vi "Dispenser Testing.vi"() -> ()   [LabVIEW 2017]
uses:
  Shared Components/Config Manager Class/Type Definitions/Potting Parameters.ctl
  Shared Components/Gantry Class/Type Definitions/Virtual Modes.ctl
  Shared Components/Gantry Class/Type Definitions/Init_Modes.ctl
  Shared Components/Config Manager Class/Type Definitions/Camera Enum.ctl
  Shared Components/WorkTable Class/Type Definitions/Worktable_Syringe.ctl
  Shared Components/Vec3d Class/Vec3d Class.lvclass
  Shared Components/Config Manager Class/Type Definitions/Potting Surface Type.ctl
  Shared Components/Gantry Class/Gantry Class.lvclass
  Shared Components/SyringeTool Class/SyringeTool Class.lvclass
  Shared Components/WorkTable Class/WorkTable Class.lvclass
panel:
  in  "Virtual Mode":T1=enum."Virtual"
  in  "Type of Potting":enum16{"Long Line", "Line", "Points"}(ring)
  in  "Potting Parameters":T2={"Curing Param A"=0.0, "Curing Param B"=0.0, "Speed Nominal"=0.5, "Time Nominal"=2.0, "Turn-on Time"=0.5, "Turn-off Time"=0.1, "Safe Height Offset"=0.0, "Tip Height"=0.18, "Width of Line"=0.0, "Number of lines"=0.0, "Distance between lines"=0.1}
  in  "stop":bool
  out "Image":T3(plugin-control)
  out "error out":errorcluster
  in  "Config Folder":path=path "C:/Users/Admin/Gantry Purdue/pixel-gantry-control/Config"
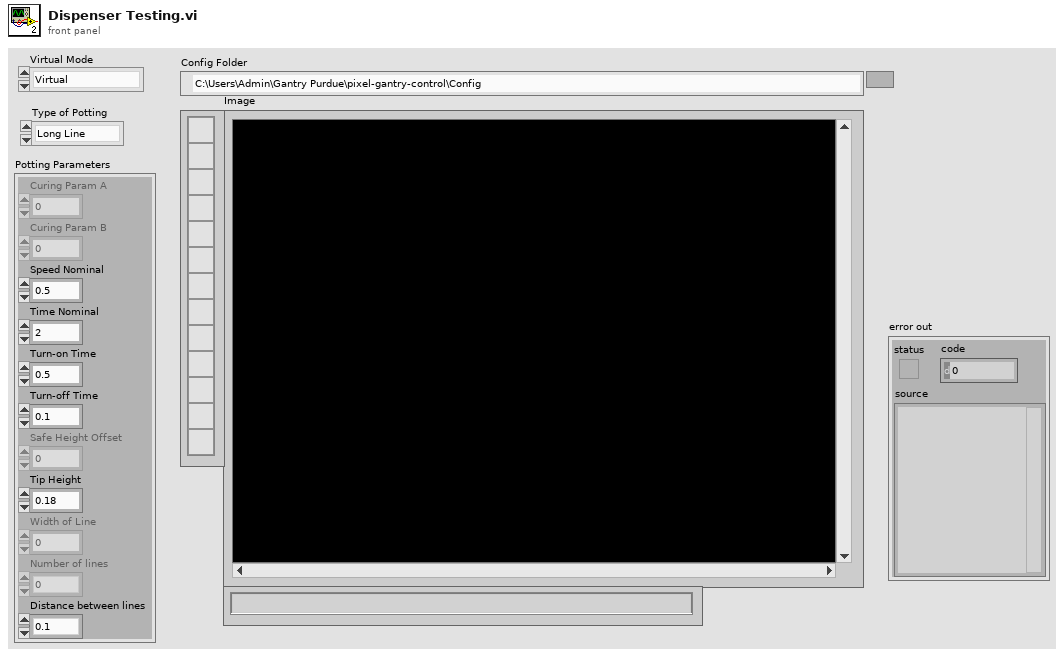
[diagram p1: front panel]
types:
  T1 = typedef "Virtual Modes.ctl" = enum16{"Nonvirtual", "Pseudovirtual", "Virtual"}
  T2 = typedef "Potting Parameters.ctl" = cluster{"Curing Param A":dbl, "Curing Param B":dbl, "Speed Nominal":dbl, "Time Nominal":dbl, "Turn-on Time":dbl, "Turn-off Time":dbl, "Safe Height Offset":dbl, "Tip Height":dbl, "Width of Line":dbl, "Number of lines":dbl, "Distance between lines":dbl}
  T3 = typedef "IMAQ Image.ctl" = refnum<image>
  T4 = typedef "Camera Enum.ctl" = enum16{"GANTRY HEAD", "NEEDLE CALIBRATION X", "NEEDLE CALIBRATION Y", "STAND CAMERA", "SIMRAN WEBCAM"}
  T5 = typedef "Init_Modes.ctl" = enum16{"Full", "Robot Only", "Dispenser Only", "Cameras Only", "Robot and Cameras", "Robot and Cameras and Dispenser", "Manifold Only"}
  T6 = typedef "Potting Surface Type.ctl" = enum16{"default", "hdi_edge_pads", "bbm_edge_pads", "address_pads"}
  T7 = typedef "Worktable_Syringe.ctl" = cluster{"Syringe Holder":enum16{"Empty", "Populated", "Calibrated"}, "Mixing Time":timestamp, "Tip Offset":refnum<class "Vec3d Class.lvclass">}
  T8 = enum16{"Left Button", "Center Button", "Right Button", "Window Close"}
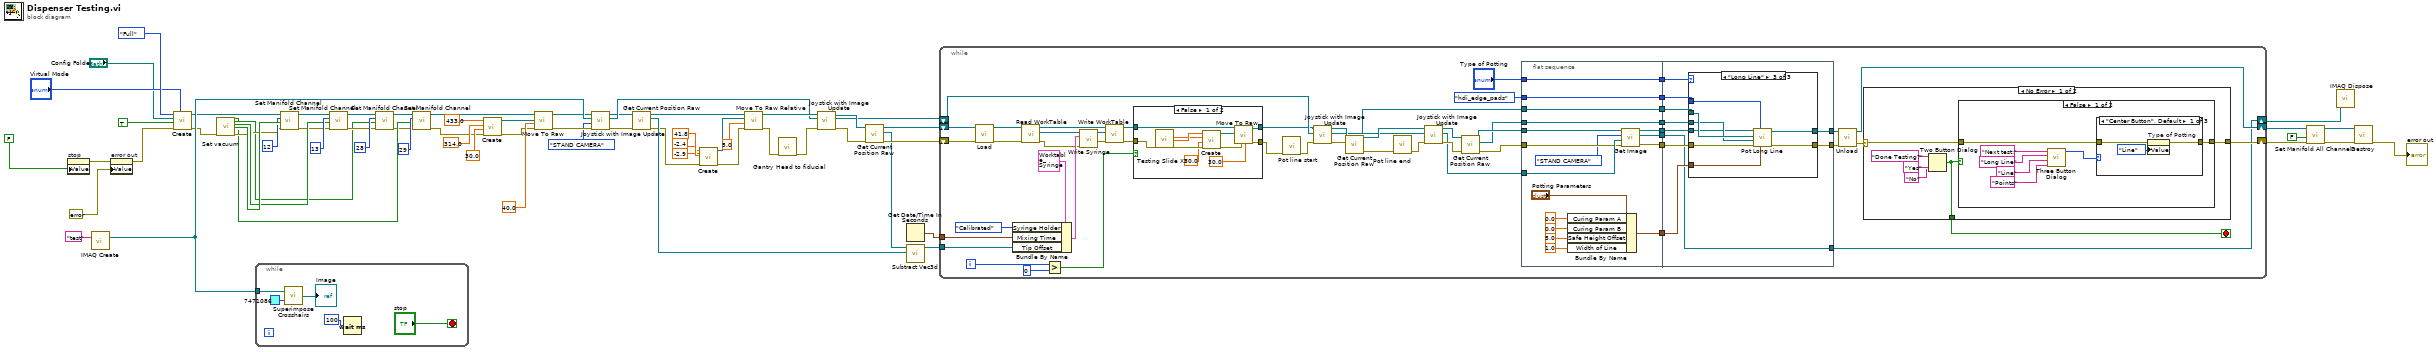
[diagram p0: block diagram]
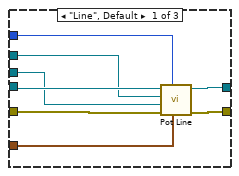
[diagram p2: hidden frame]
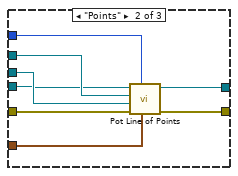
[diagram p3: hidden frame]
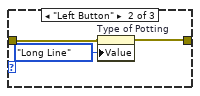
[diagram p4: hidden frame]
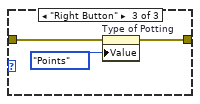
[diagram p5: hidden frame]
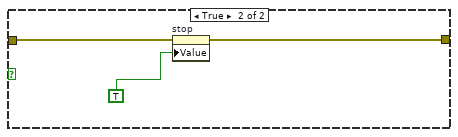
[diagram p6: hidden frame]
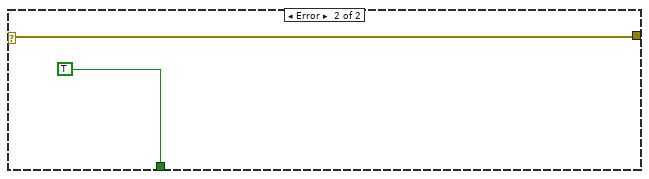
[diagram p7: hidden frame]
diagram:
  n1 = property on="stop" class="Bool (strict)"("Value"=FALSE) -> (error out=w56:errorcluster)  [unwired: 2 in, 1 out]
  n2 = call "IMAQ Create"("Image Name"="test") -> ("New Image"=w65:T3)  [unwired: 4 in, 1 out]
  n3 = property on="error out" class="Clust (strict)"(error in=w56, "Value"=errorcluster {"status"=FALSE, "code"=0, "source"=""} ("error in (no error)")) -> (error out=w55:errorcluster)  [unwired: 1 in, 1 out]
  n4 = call "Create.vi"("Virtual Mode"="Virtual Mode", "error in"=w55, "HOME?"=TRUE, "Config Folder"="Config Folder", "Init Mode"=Init_Modes."Full") -> ("error out"=w24:errorcluster, "Gantry out"=w21:refnum<class "Gantry Class.lvclass">)  [unwired: 5 in]
  n5 = call "Set vacuum"("error in (no error)"=w24) -> ("Vacuum 2B"=w8:bool, "Vacuum 2A"=w11:bool, "Vacuum 1B"=w16:bool, "Vacuum 1A"=w23:bool, "error out"=w15:errorcluster)  [unwired: 13 in, 1 out]
  n6 = while {
    tunnel: w65 -> [w71]
    stop <- "stop" stop-if-true
    n7 = call "Superimpose Crosshairs.vi"("Grid Line Color"=u32 7471086, "Refnum in"=w71) -> ("Refnum out"=→"Image":T3)
    n8 = Wait (ms)(milliseconds to wait=u32 100) -> ()  [unwired: 1 out]
  }
  n9 = call-dynamic "Set Manifold Channel.vi"("error in"=w15, "On/Off"=w23, "Manifold Channel"=12, "Gantry in"=w21) -> ("error out"=w14:errorcluster, "Gantry out"=w17:refnum<class "Gantry Class.lvclass">)  [unwired: 6 in]
  n10 = call-dynamic "Set Manifold Channel.vi"("error in"=w14, "On/Off"=w16, "Manifold Channel"=13, "Gantry in"=w17) -> ("error out"=w13:errorcluster, "Gantry out"=w12:refnum<class "Gantry Class.lvclass">)  [unwired: 6 in]
  n11 = call-dynamic "Set Manifold Channel.vi"("error in"=w13, "On/Off"=w11, "Manifold Channel"=28, "Gantry in"=w12) -> ("error out"=w7:errorcluster, "Gantry out"=w10:refnum<class "Gantry Class.lvclass">)  [unwired: 6 in]
  n12 = call-dynamic "Set Manifold Channel.vi"("error in"=w7, "On/Off"=w8, "Manifold Channel"=29, "Gantry in"=w10) -> ("error out"=w6:errorcluster, "Gantry out"=w9:refnum<class "Gantry Class.lvclass">)  [unwired: 6 in]
  n13 = call "Create.vi"("error in"=w6, "Z"=30.0, "Y"=314.0, "X"=433.0) -> ("error out"=w46:errorcluster, "Vec3d Class out"=w51:refnum<class "Vec3d Class.lvclass">)  [unwired: 6 in]
  n14 = call-dynamic "Move To Raw.vi"("error in"=w46, "Speed"=40.0, "Destination"=w51, "Gantry in"=w9) -> ("error out"=w30:errorcluster, "Gantry out"=w31:refnum<class "Gantry Class.lvclass">)  [unwired: 6 in]
  n15 = call-dynamic "Joystick with Image Update.vi"("error in (no error)"=w30, "Camera Name"=Camera_Enum."STAND CAMERA", "Image In"=w65, "Gantry Class in"=w31) -> ("error out"=w36:errorcluster, "Image Out"=w39:T3, "Gantry Class out"=w37:refnum<class "Gantry Class.lvclass">)  [unwired: 5 in]
  n16 = call-dynamic "Get Current Position Raw.vi"("error in"=w36, "Gantry in"=w37) -> ("error out"=w33:errorcluster, "Vec3d Class out"=w34:refnum<class "Vec3d Class.lvclass">, "Gantry out"=w35:refnum<class "Gantry Class.lvclass">)  [unwired: 7 in]
  n17 = call "Create.vi"("error in"=w33, "Z"=-2.9, "Y"=-2.4, "X"=41.8) -> ("error out"=w38:errorcluster, "Vec3d Class out"=w45:refnum<class "Vec3d Class.lvclass">)  [unwired: 6 in]
  n18 = call-dynamic "Move To Raw Relative.vi"("error in"=w38, "Speed(mm/s)"=5.0 ("Speed"), "Delta"=w45, "Gantry in"=w35) -> ("error out"=w40:errorcluster, "Gantry out"=w43:refnum<class "Gantry Class.lvclass">)  [unwired: 6 in]
  n19 = call "Gantry Head to fiducial"("error in (no error)"=w40) -> ("error out"=w52:errorcluster)  [unwired: 9 in, 1 out]
  n20 = call-dynamic "Joystick with Image Update.vi"("error in (no error)"=w52, "Image In"=w39, "Gantry Class in"=w43) -> ("error out"=w63:errorcluster, "Image Out"=w58:T3, "Gantry Class out"=w64:refnum<class "Gantry Class.lvclass">)  [unwired: 6 in]
  n21 = call-dynamic "Get Current Position Raw.vi"("error in"=w63, "Gantry in"=w64) -> ("error out"=w61:errorcluster, "Vec3d Class out"=w57:refnum<class "Vec3d Class.lvclass">, "Gantry out"=w62:refnum<class "Gantry Class.lvclass">)  [unwired: 7 in]
  n22 = Get Date/Time In Seconds() -> (seconds since 1Jan1904=w59:timestamp)
  n23 = call "Subtract Vec3d.vi"("Vec3d in 2"=w34, "Vec3d in 1"=w57) -> ("Vec3d Class out"=w60:refnum<class "Vec3d Class.lvclass">)  [unwired: 8 in, 1 out]
  n24 = while {
    tunnel: w60 -> [w118]
    tunnel: w59 -> [w117]
    shift-right: [w74] -> w53
    shift-left: w58 -> [w107]
    shift-right: [w77] -> w5
    shift-left: w62 -> [w126]
    shift-right: [w98] -> w4
    shift-left: w61 -> [w125]
    i -> [w91]
    stop <- w86 stop-if-true
    n25 = call "Load.vi"("error in"=w125, "Gantry in"=w126) -> ("error out"=w123:errorcluster, "SyringeTool out"=w124:refnum<class "SyringeTool Class.lvclass">)  [unwired: 8 in]
    n26 = Bundle By Name(cluster=T7 {"Syringe Holder"=enum."Empty", "Mixing Time"=timestamp(0 s since 1904-01-01), "Tip Offset"=refnum} ("Syringe"), "Syringe Holder"=enum16{"Empty", "Populated", "Calibrated"}."Calibrated", "Mixing Time"=w117, "Tip Offset"=w118) -> (w120:T7)
    n27 = call-dynamic "Read WorkTable.vi"("error in"=w123, "Gantry Class in"=w124) -> ("error out"=w114:errorcluster, "WorkTable Class.lvclass"=w122:refnum<class "WorkTable Class.lvclass">, "Gantry Class out"=w116:refnum<class "SyringeTool Class.lvclass">)  [unwired: 7 in]
    n28 = Greater?(x=w91, y=0) -> (0:w89:bool)
    n29 = call-dynamic "Write Syringe.vi"("error in (no error)"=w114, "Syringe"=w120, "WorkTable Class in"=w122) -> ("error out"=w113:errorcluster, "WorkTable Class out"=w115:refnum<class "WorkTable Class.lvclass">)  [unwired: 7 in]
    n30 = call-dynamic "Write WorkTable.vi"("error in (no error)"=w113, "WorkTable Class.lvclass"=w115, "Gantry Class in"=w116) -> ("error out"=w94:errorcluster, "Gantry Class out"=w93:refnum<class "SyringeTool Class.lvclass">)  [unwired: 7 in]
    n31 = case shown="False" w89 {
      tunnel: w94 -> [w209 w216]
      tunnel: w93 -> [w208 w217]
      tunnel: [w207 w216] -> w92
      tunnel: [w205 w217] -> w88
      frame False {
        n32 = call "Testing Slide XY"("error in (no error)"=w209) -> ("Y"=w214:dbl, "X"=w215:dbl, "error out"=w210:errorcluster)  [unwired: 15 in, 1 out]
        n33 = call "Create.vi"("error in"=w210, "Z"=30.0, "Y"=w214, "X"=w215) -> ("error out"=w211:errorcluster, "Vec3d Class out"=w213:refnum<class "Vec3d Class.lvclass">)  [unwired: 6 in]
        n34 = call-dynamic "Move To Raw.vi"("error in"=w211, "Speed"=30.0, "Destination"=w213, "Gantry in"=w208) -> ("error out"=w207:errorcluster, "Gantry out"=w205:refnum<class "SyringeTool Class.lvclass">)  [unwired: 6 in]
      }
      frame True {
      }
    }
    n35 = call "Pot line start"("error in (no error)"=w92) -> ("error out"=w97:errorcluster)  [unwired: 9 in, 1 out]
    n36 = call-dynamic "Joystick with Image Update.vi"("error in (no error)"=w97, "Image In"=w107, "Gantry Class in"=w88) -> ("error out"=w100:errorcluster, "Image Out"=w110:T3, "Gantry Class out"=w112:refnum<class "SyringeTool Class.lvclass">)  [unwired: 6 in]
    n37 = call-dynamic "Get Current Position Raw.vi"("error in"=w100, "Gantry in"=w112) -> ("error out"=w96:errorcluster, "Vec3d Class out"=w105:refnum<class "Vec3d Class.lvclass">, "Gantry out"=w111:refnum<class "SyringeTool Class.lvclass">)  [unwired: 7 in]
    n38 = call "Pot line end"("error in (no error)"=w96) -> ("error out"=w95:errorcluster)  [unwired: 9 in, 1 out]
    n39 = call-dynamic "Joystick with Image Update.vi"("error in (no error)"=w95, "Image In"=w110, "Gantry Class in"=w111) -> ("error out"=w108:errorcluster, "Image Out"=w76:T3, "Gantry Class out"=w109:refnum<class "SyringeTool Class.lvclass">)  [unwired: 6 in]
    n40 = call-dynamic "Get Current Position Raw.vi"("error in"=w108, "Gantry in"=w109) -> ("error out"=w101:errorcluster, "Vec3d Class out"=w104:refnum<class "Vec3d Class.lvclass">, "Gantry out"=w106:refnum<class "SyringeTool Class.lvclass">)  [unwired: 7 in]
    n41 = flat-sequence {
      tunnel: w101 -> [w130]
      tunnel: Potting_Surface_Type."hdi_edge_pads" ("Potting Surface Type") -> [w141]
      tunnel: w104 -> [w142]
      tunnel: w105 -> [w143]
      tunnel: w106 -> [w132]
      tunnel: [w131] -> w85
      tunnel: [w143] -> w84
      tunnel: [w142] -> w83
      tunnel: [w141] -> w82
      tunnel: [w129] -> w81
      tunnel: [w139] -> w80
      tunnel: [w134] -> w79
      tunnel: "Type of Potting" -> [w134]
      tunnel: w76 -> [w133]
      tunnel: [w127] -> w75
      tunnel: [w149] -> w102
      tunnel: [w147] -> w99
      tunnel: w85 -> [w153]
      tunnel: w84 -> [w152]
      tunnel: w83 -> [w151]
      tunnel: w82 -> [w150]
      tunnel: w81 -> [w148]
      tunnel: w80 -> [w146]
      tunnel: w79 -> [w145]
      tunnel: [w144] -> w74
      tunnel: w75 -> [w144]
      frame #0 {
        n42 = Bundle By Name(cluster="Potting Parameters", "Curing Param A"=0.0, "Curing Param B"=0.0, "Safe Height Offset"=5.0, "Width of Line"=1.0 ("Pot Length Scale")) -> (w139:T2)
        n43 = call-dynamic "Get Image.vi"("error in"=w130, "Image In"=w133, "Camera Name"=Camera_Enum."STAND CAMERA", "Gantry in"=w132) -> ("error out"=w129:errorcluster, "Image Out"=w127:T3, "Gantry out"=w131:refnum<class "SyringeTool Class.lvclass">)  [unwired: 4 in, 1 out]
      }
      frame #1 {
        n44 = case shown="\"Long Line\"" w145 {
          tunnel: w153 -> [w161 w164 w174]
          tunnel: w152 -> [w160 w168 w176]
          tunnel: w151 -> [w159 w167 w175]
          tunnel: w150 -> [w158 w169 w177]
          tunnel: [w157 w165 w173] -> w149
          tunnel: w148 -> [w155 w163 w172]
          tunnel: [w156 w166 w171] -> w147
          tunnel: w146 -> [w154 w162 w170]
          frame "Line", Default {
            n45 = call-dynamic "Pot Line.vi"("Potting Parameters"=w154, "Potting Surface Type"=w158, "error in"=w155, "End Position"=w159, "Start Position"=w160, "SyringeTool in"=w161) -> ("error out"=w156:errorcluster, "SyringeTool out"=w157:refnum<class "SyringeTool Class.lvclass">)  [unwired: 4 in]
          }
          frame "Points" {
            n46 = call-dynamic "Pot Line of Points.vi"("Potting Parameters"=w162, "Potting Surface Type"=w169, "error in (no error)"=w163, "End Position"=w167, "Start Position"=w168, "SyringeTool Class in"=w164) -> ("error out"=w166:errorcluster, "SyringeTool Class out"=w165:refnum<class "SyringeTool Class.lvclass">)  [unwired: 4 in]
          }
          frame "Long Line" {
            n47 = call-dynamic "Pot Long Line.vi"("Potting Parameters"=w170, "Potting Surface Type"=w177, "error in"=w172, "End Position"=w175, "Start Position"=w176, "SyringeTool in"=w174) -> ("error out"=w171:errorcluster, "SyringeTool out"=w173:refnum<class "SyringeTool Class.lvclass">)  [unwired: 4 in]
          }
        }
      }
    }
    n48 = call "Unload.vi"("error in"=w99, "SyringeTool in"=w102) -> ("error out"=w87:errorcluster, "Gantry out"=w77:refnum<class "Gantry Class.lvclass">)  [unwired: 8 in]
    n49 = case shown="No Error" w87 {
      selector: w87 -> [w179 w204]
      tunnel: [w178 w204] -> w98
      tunnel: [w180 TRUE ("Done Testing?")] -> w86
      frame No Error {
        n50 = Two Button Dialog(message="Done Testing?", 1:"No" ("F button name (\"Cancel\")"), 2:"Yes" ("T button name (\"OK\")")) -> (T button?=w180:bool)
        n51 = case shown="False" w180 {
          tunnel: w179 -> [w189 w202]
          tunnel: [w188 w200] -> w178
          frame False {
            n52 = call <vilib>:"Three Button Dialog.vi"("Right Button Text (\"Cancel\")"="Points" ("F button name (\"Cancel\")"), "Center Button Text (\"No\")"="Line" ("T button name (\"OK\")"), "Left Button Text (\"Yes\")"="Long Line" ("T button name (\"OK\")"), "message"="Next test:") -> ("Which Button?"=w190:T8)  [unwired: 7 in]
            n53 = case shown="\"Center Button\", Default" w190 {
              tunnel: w189 -> [w193 w196 w198]
              tunnel: [w192 w195 w197] -> w188
              frame "Center Button", Default {
                n54 = property on="Type of Potting" class="Enum (strict)"(error in=w193, "Value"=enum16{"Long Line", "Line", "Points"}."Line" ("Type of Potting")) -> (error out=w192:errorcluster)  [unwired: 1 in, 1 out]
              }
              frame "Left Button" {
                n55 = property on="Type of Potting" class="Enum (strict)"(error in=w196, "Value"=enum16{"Long Line", "Line", "Points"}."Long Line" ("Type of Potting")) -> (error out=w195:errorcluster)  [unwired: 1 in, 1 out]
              }
              frame "Right Button" {
                n56 = property on="Type of Potting" class="Enum (strict)"(error in=w198, "Value"=enum16{"Long Line", "Line", "Points"}."Points" ("Type of Potting")) -> (error out=w197:errorcluster)  [unwired: 1 in, 1 out]
              }
            }
          }
          frame True {
            n57 = property on="stop" class="Bool (strict)"(error in=w202, "Value"=TRUE) -> (error out=w200:errorcluster)  [unwired: 1 in, 1 out]
          }
        }
      }
      frame Error {
      }
    }
  }
  n58 = call-dynamic "Set Manifold All Channels.vi"("error in"=w4, "On/Off"=FALSE, "Gantry in"=w5) -> ("error out"=w2:errorcluster, "Gantry out"=w3:refnum<class "Gantry Class.lvclass">)  [unwired: 7 in]
  n59 = call "IMAQ Dispose"("Image"=w53) -> ()  [unwired: 5 in, 1 out]
  n60 = call "Destroy.vi"("error in"=w2, "Gantry Class in"=w3) -> ("error out"=→"error out":errorcluster)  [unwired: 9 in]
